vi "Shift_Logic.vi"(8 "error in (no error)":errorcluster, 11 "Time Stamp IN":timestamp[](array[timestamp]) format="%<%X>T") -> (0 "error out":errorcluster, 3 "Shift":i32)   [LabVIEW 2017]
panel:
  out "double precision float":dbl format="%#_13g"
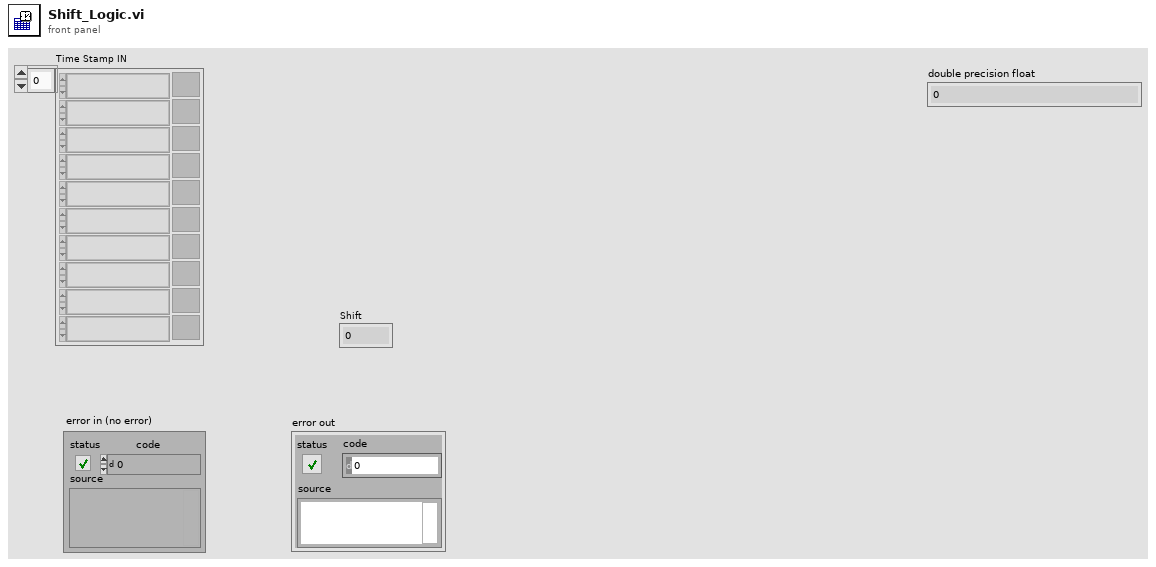
[diagram p1: front panel]
types:
  T1 = typedef "LVDateTimeRec.ctl" = cluster{"fractional second":dbl, "second":i32, "minute":i32, "hour":i32, "day of month":i32, "month":i32, "year":i32, "day of week":i32, "day of year":i32, "DST":i32}
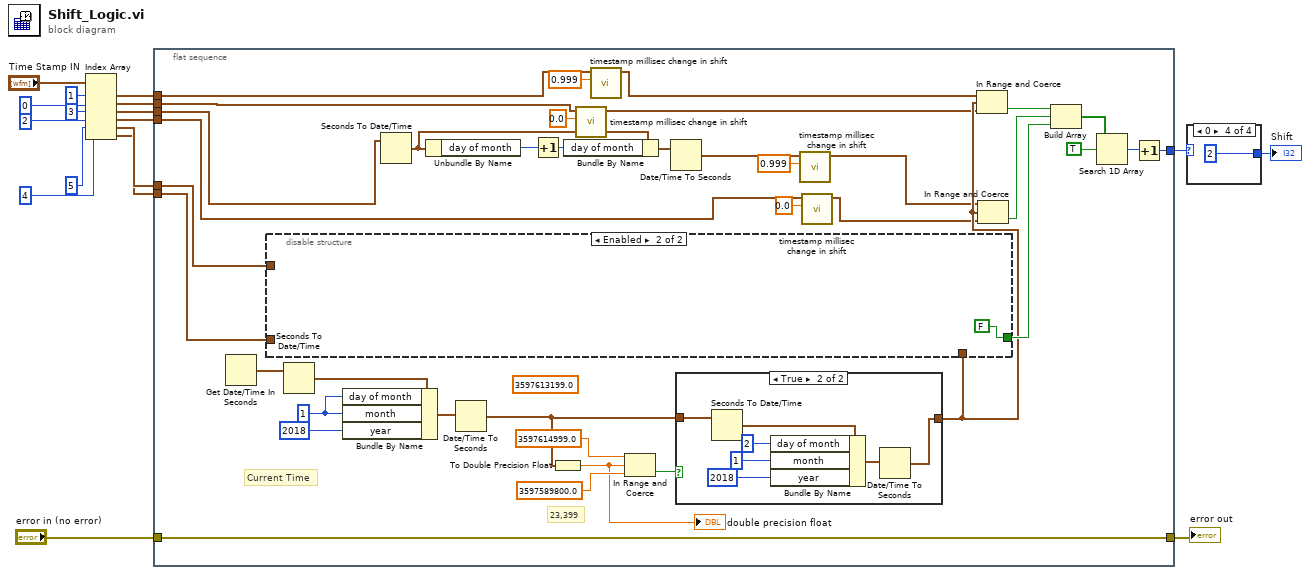
[diagram p0: block diagram]
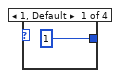
[diagram p2: hidden frame]
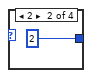
[diagram p3: hidden frame]
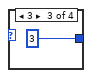
[diagram p4: hidden frame]
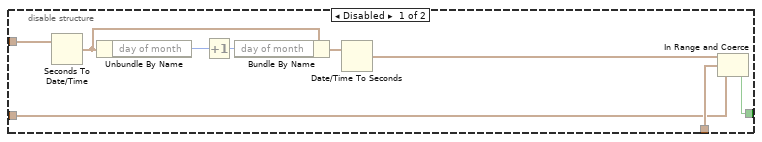
[diagram p5: hidden frame]
diagram:
  n1 = Index Array(array="Time Stamp IN", index #1=1 ("index"), index #2=0 ("index"), index #3=3 ("index"), index #4=2 ("index"), index #5=5 ("index"), index #6=4 ("index")) -> (element #1=w14:timestamp, element #2=w13:timestamp, element #3=w10:timestamp, element #4=w9:timestamp, element #5=w6:timestamp, element #6=w5:timestamp)
  n2 = flat-sequence {
    tunnel: [w49] -> w4
    tunnel: "error in (no error)" -> [w38]
    tunnel: [w38] -> w1
    tunnel: w14 -> [w29]
    tunnel: w13 -> [w25]
    tunnel: w10 -> [w30]
    tunnel: w9 -> [w20]
    tunnel: w6 -> [w37]
    tunnel: w5 -> [w36]
    frame #0 {
      (unwired) 3597613199.0 ("double precision float 2")
      w42 = 1 ("day of month")
      # "Current Time"
      # "23,399"
      n3 = Get Date/Time In Seconds() -> (seconds since 1Jan1904=w35:timestamp)
      n4 = Seconds To Date/Time(time stamp (now)=w35) -> (date time rec=w46:T1)  [unwired: 1 in]
      n5 = Bundle By Name(cluster=w46, "day of month"=w42, "month"=w42, "year"=2018) -> (w48:T1)
      n6 = Seconds To Date/Time(time stamp (now)=w30) -> (date time rec=w33:T1)  [unwired: 1 in]
      n7 = Unbundle By Name(w33) -> ("day of month"=w31:i32)
      n8 = Date/Time To Seconds(2:w48) -> (0:w40:timestamp)  [unwired: 1 in]
      n9 = Increment(x=w31) -> (x+1=w32:i32)
      n10 = To Double Precision Float(number=w40) -> (double precision float=w43:dbl)
      "double precision float" <- w43
      n11 = Bundle By Name(cluster=w33, "day of month"=w32) -> (w34:T1)
      n12 = call "timestamp millisec change in shift.vi"("fractional second"=0.0, "time stamp in"=w25) -> ("time stamp out"=w24:timestamp)  [unwired: 9 in]
      n13 = call "timestamp millisec change in shift.vi"("fractional second"=0.999, "time stamp in"=w29) -> ("time stamp out"=w28:timestamp)  [unwired: 9 in]
      n14 = In Range and Coerce(upper limit=3597614999.0 ("double precision float 2"), x=w43, lower limit=3597589800.0 ("double precision float")) -> (In Range?=w41:bool)  [unwired: 1 out]
      n15 = Date/Time To Seconds(2:w34) -> (0:w23:timestamp)  [unwired: 1 in]
      n16 = case shown="True" w41 {
        tunnel: w40 -> [w66 w69]
        tunnel: [w66 w68] -> w39
        frame False {
        }
        frame True {
          n17 = Seconds To Date/Time(time stamp (now)=w69) -> (date time rec=w71:T1)  [unwired: 1 in]
          n18 = Bundle By Name(cluster=w71, "day of month"=2, "month"=1 ("day of month"), "year"=2018) -> (w73:T1)
          n19 = Date/Time To Seconds(2:w73) -> (0:w68:timestamp)  [unwired: 1 in]
        }
      }
      n20 = disable-structure shown="Enabled" {
        disable-tunnel: [w63 FALSE] -> w53
        disable-tunnel: w39 -> [w62 _]
        disable-tunnel: w37 -> [w61 _]
        disable-tunnel: w36 -> [w60 _]
        frame Disabled {
          n21 = Seconds To Date/Time(time stamp (now)=w61) -> (date time rec=w58:T1)  [unwired: 1 in]
          n22 = Unbundle By Name(w58) -> ("day of month"=w56:i32)
          n23 = Increment(x=w56) -> (x+1=w57:i32)
          n24 = Bundle By Name(cluster=w58, "day of month"=w57) -> (w59:T1)
          n25 = Date/Time To Seconds(2:w59) -> (0:w64:timestamp)  [unwired: 1 in]
          n26 = In Range and Coerce(upper limit=w64, x=w62, lower limit=w60) -> (In Range?=w63:bool)  [unwired: 1 out]
        }
        frame Enabled {
        }
      }
      n27 = call "timestamp millisec change in shift.vi"("fractional second"=0.999, "time stamp in"=w23) -> ("time stamp out"=w22:timestamp)  [unwired: 9 in]
      n28 = call "timestamp millisec change in shift.vi"("fractional second"=0.0, "time stamp in"=w20) -> ("time stamp out"=w19:timestamp)  [unwired: 9 in]
      n29 = In Range and Coerce(upper limit=w28, x=w39, lower limit=w24) -> (In Range?=w55:bool)  [unwired: 1 out]
      n30 = In Range and Coerce(upper limit=w22, x=w39, lower limit=w19) -> (In Range?=w54:bool)  [unwired: 1 out]
      n31 = Build Array(w55, w54, w53) -> (w52:bool[])
      n32 = Search 1D Array(1D array=w52, element=TRUE) -> (index of element=w50:i32)  [unwired: 1 in]
      n33 = Increment(x=w50) -> (x+1=w49:i32)
    }
  }
  n34 = case shown="0" w4 {
    tunnel: [1 2 3 2] -> w3
    frame 1, Default {
    }
    frame 2 {
    }
    frame 3 {
    }
    frame 0 {
    }
  }
  "Shift" <- w3
  "error out" <- w1
